vi "updateDeviceStatus.vi"(0 "OrionBMS in":refnum<class "OrionBMSClass.lvclass">, 1 "isNewData":bool, 3 "error in (no error)":errorcluster) -> (7 "OrionBMS out":refnum<class "OrionBMSClass.lvclass">, 10 "error out":errorcluster)   [LabVIEW 2018, in "OrionBMSClass.lvclass"]
uses:
  OrionBMSClass.lvclass
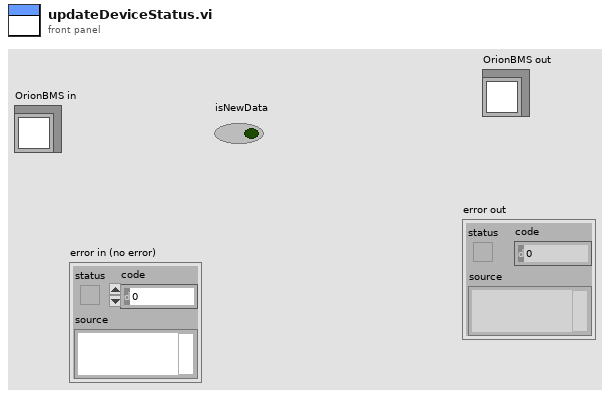
[diagram p1: front panel]
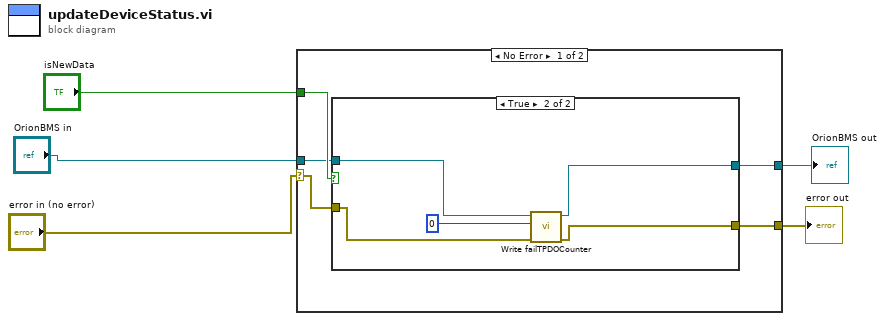
[diagram p0: block diagram]
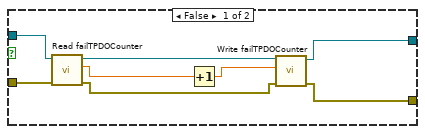
[diagram p2: hidden frame]
diagram:
  n1 = case shown="No Error" "error in (no error)" {
    selector: "error in (no error)" -> [w7 w24]
    tunnel: "isNewData" -> [w10 _]
    tunnel: "OrionBMS in" -> [w9 w25]
    tunnel: [w8 w25] -> w3
    tunnel: [w6 w24] -> w1
    frame No Error {
      n2 = case shown="True" w10 {
        tunnel: w9 -> [w16 w22]
        tunnel: [w14 w20] -> w8
        tunnel: w7 -> [w13 w21]
        tunnel: [w11 w19] -> w6
        frame False {
          n3 = call-dynamic "Read failTPDOCounter.vi"("error in (no error)"=w13, "OrionBMS in"=w16) -> ("error out"=w12:errorcluster, "failTPDOCounter"=w18:dbl, "OrionBMS out"=w15:refnum<class "OrionBMSClass.lvclass">)  [unwired: 7 in]
          n4 = Increment(x=w18) -> (x+1=w17:dbl)
          n5 = call-dynamic "Write failTPDOCounter.vi"("error in (no error)"=w12, "failTPDOCounter"=w17, "OrionBMS in"=w15) -> ("error out"=w11:errorcluster, "OrionBMS out"=w14:refnum<class "OrionBMSClass.lvclass">)  [unwired: 7 in]
        }
        frame True {
          n6 = call-dynamic "Write failTPDOCounter.vi"("error in (no error)"=w21, "failTPDOCounter"=u8 0, "OrionBMS in"=w22) -> ("error out"=w19:errorcluster, "OrionBMS out"=w20:refnum<class "OrionBMSClass.lvclass">)  [unwired: 7 in]
        }
      }
    }
    frame Error {
    }
  }
  "OrionBMS out" <- w3
  "error out" <- w1
